vi "CPU_MEM_initialize_ROMs.vi"(8 "error in (no error)":errorcluster) -> (0 "error out":errorcluster)   [LabVIEW 2018]
uses:
  CPU_MEM_references.vi
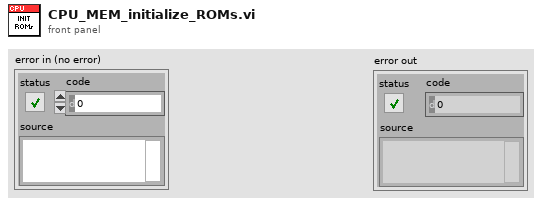
[diagram p1: front panel]
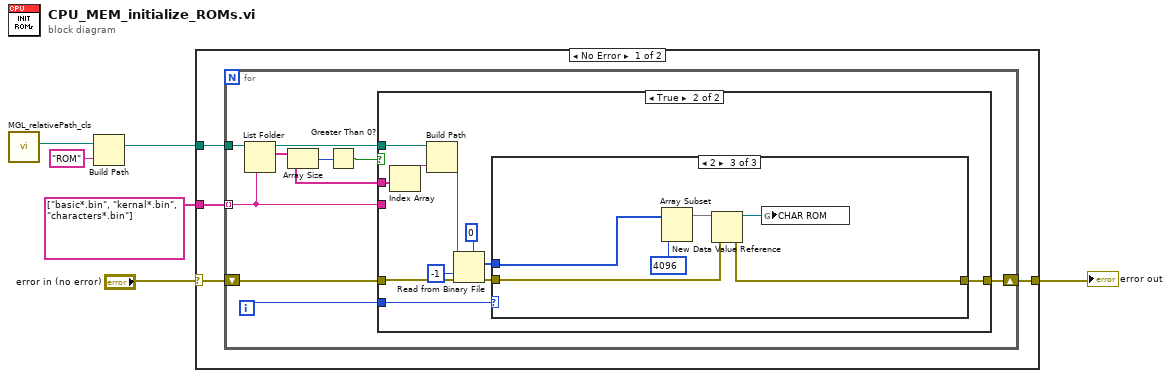
[diagram p0: block diagram]
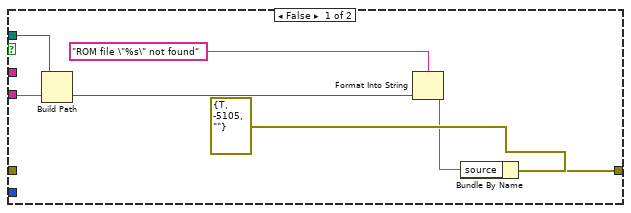
[diagram p2: hidden frame]
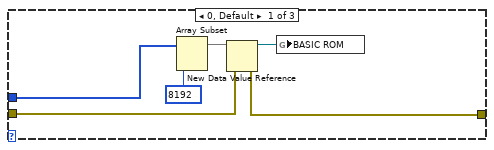
[diagram p3: hidden frame]
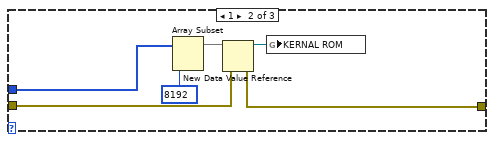
[diagram p4: hidden frame]
diagram:
  n1 = call "MGL_relativePath_cls.vi"() -> ("Path"=w6:path)  [unwired: 8 in, 1 out]
  n2 = Build Path(base path=w6, name or relative path="ROM") -> (appended path=w4:path)
  n3 = case shown="No Error" "error in (no error)" {
    selector: "error in (no error)" -> [w8 w56]
    tunnel: w4 -> [w10 _]
    tunnel: string[] ["basic*.bin", "kernal*.bin", "characters*.bin"] -> [w9 _]
    tunnel: [w7 w56] -> w1
    frame No Error {
      n4 = for {
        tunnel: w10 -> [w19]
        tunnel: w9 -> [w16] mode=indexing
        shift-right: [w14] -> w7
        shift-left: w8 -> [w13]
        i -> [w11]
        n5 = List Folder(path=w19, pattern=w16) -> (path out=w15:path, filenames=w12:string[])  [unwired: 2 in, 2 out]
        n6 = Array Size(array=w12) -> (size(s)=w18:i32)
        n7 = Greater Than 0?(x=w18) -> (x > 0?=w17:bool)
        n8 = case shown="True" w17 {
          tunnel: w16 -> [w25 _]
          tunnel: w15 -> [w24 w34]
          tunnel: [w21 w27] -> w14
          tunnel: w13 -> [_ w35]
          tunnel: w12 -> [_ w33]
          tunnel: w11 -> [_ w30]
          frame False {
            n9 = Build Path(base path=w24, name or relative path=w25) -> (appended path=w23:path)
            n10 = Format Into String(format string="ROM file \"%s\" not found", w23) -> (resulting string=w20:string)  [unwired: 2 in, 1 out]
            n11 = Bundle By Name(cluster=errorcluster {"status"=TRUE, "code"=-5105, "source"=""} ("error out"), "source"=w20) -> (w21:errorcluster)
          }
          frame True {
            n12 = Index Array(array=w33) -> (element=w32:string)  [unwired: 1 in]
            n13 = Build Path(base path=w34, name or relative path=w32) -> (appended path=w31:path)
            n14 = Read from Binary File(5:u8 0 ("data type"), 8:w35, 10:-1 ("count (1)"), 11:w31) -> (0:w28:errorcluster, 2:w29:u8[])  [unwired: 2 in, 2 out]
            n15 = case shown="2" w30 {
              tunnel: w29 -> [w40 w47 w52]
              tunnel: w28 -> [w39 w45 w51]
              tunnel: [w38 w44 w50] -> w27
              frame 0, Default {
                n16 = Array Subset(array=w40, length=8192) -> (w42:u8[])  [unwired: 1 in]
                n17 = New Data Value Reference(data value=w42, error in=w39) -> (data value reference=w43:refnum<data-value>, error out=w38:errorcluster)
                n18 = global write "CPU_MEM_references.vi" "BASIC ROM"(w43) -> ()
              }
              frame 1 {
                n19 = Array Subset(array=w47, length=8192) -> (w48:u8[])  [unwired: 1 in]
                n20 = New Data Value Reference(data value=w48, error in=w45) -> (data value reference=w49:refnum<data-value>, error out=w44:errorcluster)
                n21 = global write "CPU_MEM_references.vi" "KERNAL ROM"(w49) -> ()
              }
              frame 2 {
                n22 = Array Subset(array=w52, length=4096) -> (w54:u8[])  [unwired: 1 in]
                n23 = New Data Value Reference(data value=w54, error in=w51) -> (data value reference=w55:refnum<data-value>, error out=w50:errorcluster)
                n24 = global write "CPU_MEM_references.vi" "CHAR ROM"(w55) -> ()
              }
            }
          }
        }
      }
    }
    frame Error {
    }
  }
  "error out" <- w1
